vi "Write Excel Data.vi"(8 "error in (no error)":errorcluster, 10 "Excel Data":T1[](array[typedef]), 11 "NI Generic Parser in":refnum<class "NI Generic Parser.lvclass">) -> (0 "error out":errorcluster, 3 "NI Generic Parser out":refnum<class "NI Generic Parser.lvclass">)   [LabVIEW 2016, in "NI Generic Parser.lvlib" / "NI Generic Parser.lvclass"]
uses:
  NI Generic Parser.lvclass
  Controls/WorkSheet Data.ctl
  NI Generic Parser.lvclass/NI Generic Parser.ctl
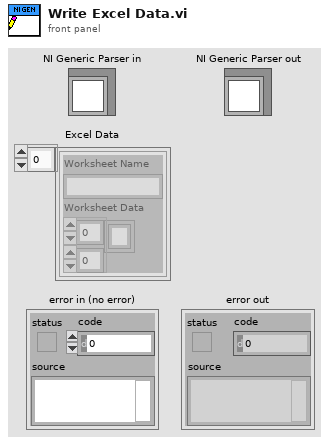
[diagram p1: front panel]
types:
  T1 = typedef "NI Generic Parser.lvlib/NI Generic Parser.lvclass/WorkSheet Data.ctl" = cluster{"Worksheet Name":string, "Worksheet Data":string[][]}
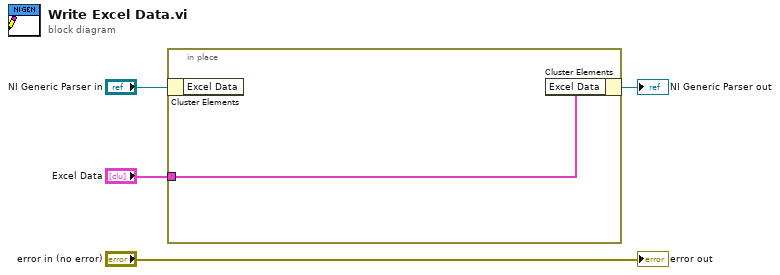
[diagram p0: block diagram]
diagram:
  n1 = in-place {
    in-place-border: "Excel Data" -> [w5]
    n2 = in-place-cluster #1("NI Generic Parser in") -> ()  [unwired: 1 out]
    n3 = in-place-cluster #1("Excel Data"=w5) -> (→"NI Generic Parser out":refnum<class "NI Generic Parser.lvclass">)
  }
  "error out" <- "error in (no error)"
